vi "mm2time001.vi"(1 "reverse?":bool, 2 "Offset (mm)":dbl, 3 "distance (mm)":dbl) -> (0 "time in fs":dbl)   [LabVIEW 2020]
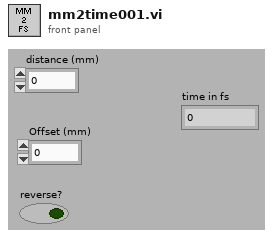
[diagram p1: front panel]
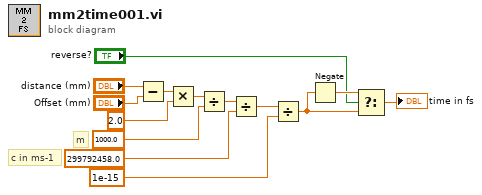
[diagram p0: block diagram]
diagram:
  # "c in ms-1"
  # "m"
  n1 = Subtract(x="distance (mm)", y="Offset (mm)") -> (x-y=w7:dbl)
  n2 = Multiply(x=w7, y=2.0) -> (x*y=w9:dbl)
  n3 = Divide(x=w9, y=1000.0) -> (x/y=w11:dbl)
  n4 = Divide(x=w11, y=299792458.0) -> (x/y=w6:dbl)
  n5 = Divide(x=w6, y=1e-15) -> (x/y=w1:dbl)
  n6 = Negate(x=w1) -> (-x=w4:dbl)
  n7 = Select(t=w4, s="reverse?", f=w1) -> (s? t:f=→"time in fs":dbl)
